vi "Workspace_test.vi"() -> ()   [LabVIEW 2017]
uses:
  NationalInstruments.VeriStand.SystemStorageUI
  NationalInstruments.VeriStand.SystemStorage
  <vilib>/NI Veristand/Execution/Workspace/NI VeriStand - Get Multiple Channel Values.vi
  <vilib>/NI Veristand/Execution/Workspace/NI_VS Workspace ExecutionAPI.lvlib
  <vilib>/NI Veristand/UI Controls/Single Node Browser/NI_VS UI Single Node Browser.lvlib
panel:
  in  "Stop":bool
  in  "NIVS.System Definition Root":refnum<k24>
  in  "Tree Browser":refnum<k24>(container)
  in  "NIVS.Project File Path":path
  in  "Single Node Browser":refnum<k24>(container)
  in  "NIVS.Workspace Event":refnum<event-registration>
  out "System Times":dbl[](array[numeric]) format="%<%H:%M:%S%3u>t"
  out "Targets":string[](array[string])
  in  "NIVS.Gateway IP Address":string
  in  "NIVS.INI File Path":path
  # "Use this example as a template to create custom tools for the NI VeriStand Workspace. This example shows the use of the NI VeriStand API and UI controls to set and get data.\n\nRun this example by adding this VI as a Workspace Tool item. For Help adding Workspace Tool items, please reference the NI VeriStand Help."
  # "With the assistance of the NI VeriStand Execution API, a tool has access to streaming data running on the target."
  # "This is the file path to the VeriStand system definition file. You can read or write to the file using the System Definition API."
  # "This is the root reference to the active System Definition file. You could use this to read the configuration or populate a tree with channels. You are free to close this reference, but it will be closed for you if you don't."
  # "The SystemStorageUI .NET assembly provides controls to display data configured in the System Definition file."
  # "This is the IP Address of the VeriStand Gateway to which the Workspace is connected. Use this to open all the .NET Manager references. Usually the Gateway is running on localhost, but it could be running on a neighbor's machine."
  # "This registered string User Event is used to help instruct your tool to shut down when the Workspace is closing."
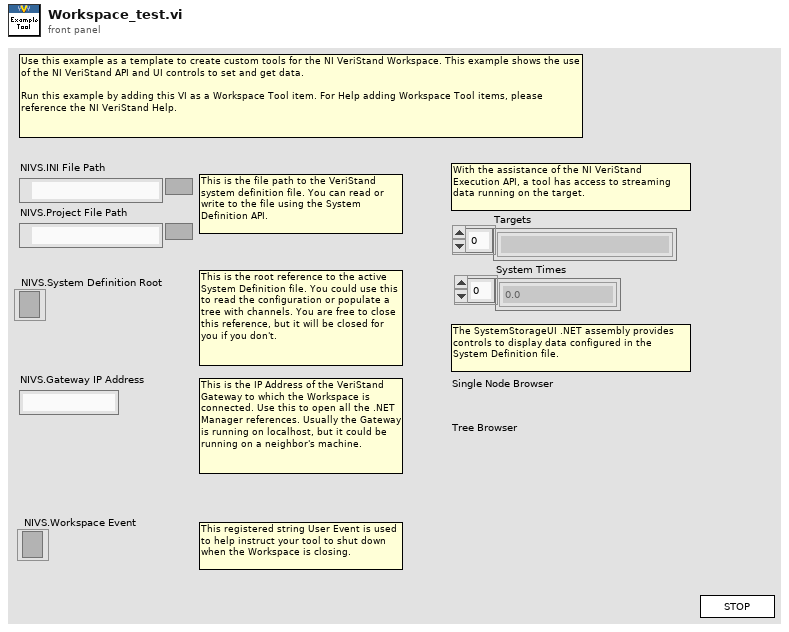
[diagram p1: front panel]
types:
  T1 = typedef "NI_VS UI Single Node Browser.lvlib/Callback Type.ctl" = cluster{"Net Callbacks":refnum<k27>[], "Event":refnum<user-event>}
  T2 = typedef "NI_VS Workspace ExecutionAPI.lvlib/WorkspaceAPI.ctl" = refnum<k24>
  T3 = typedef "NI_VS Workspace ExecutionAPI.lvlib/SystemStateEventRef.ctl" = cluster{"CustDatRef":refnum<user-event>, "EvtRef":refnum<k27>, "Target State User Event":refnum<user-event>}
  T4 = typedef "NI_VS Workspace ExecutionAPI.lvlib/SystemStateRegEventRef.ctl" = refnum<event-registration>
  T5 = cluster{"NIVS.Workspace Event":refnum<event-registration>, "Event Registration Refnum":refnum<event-registration>, "SystemChangeEventRef":T4}
  T6 = typedef "NI_VS UI Single Node Browser.lvlib/Node Ref.ctl" = refnum<k24>
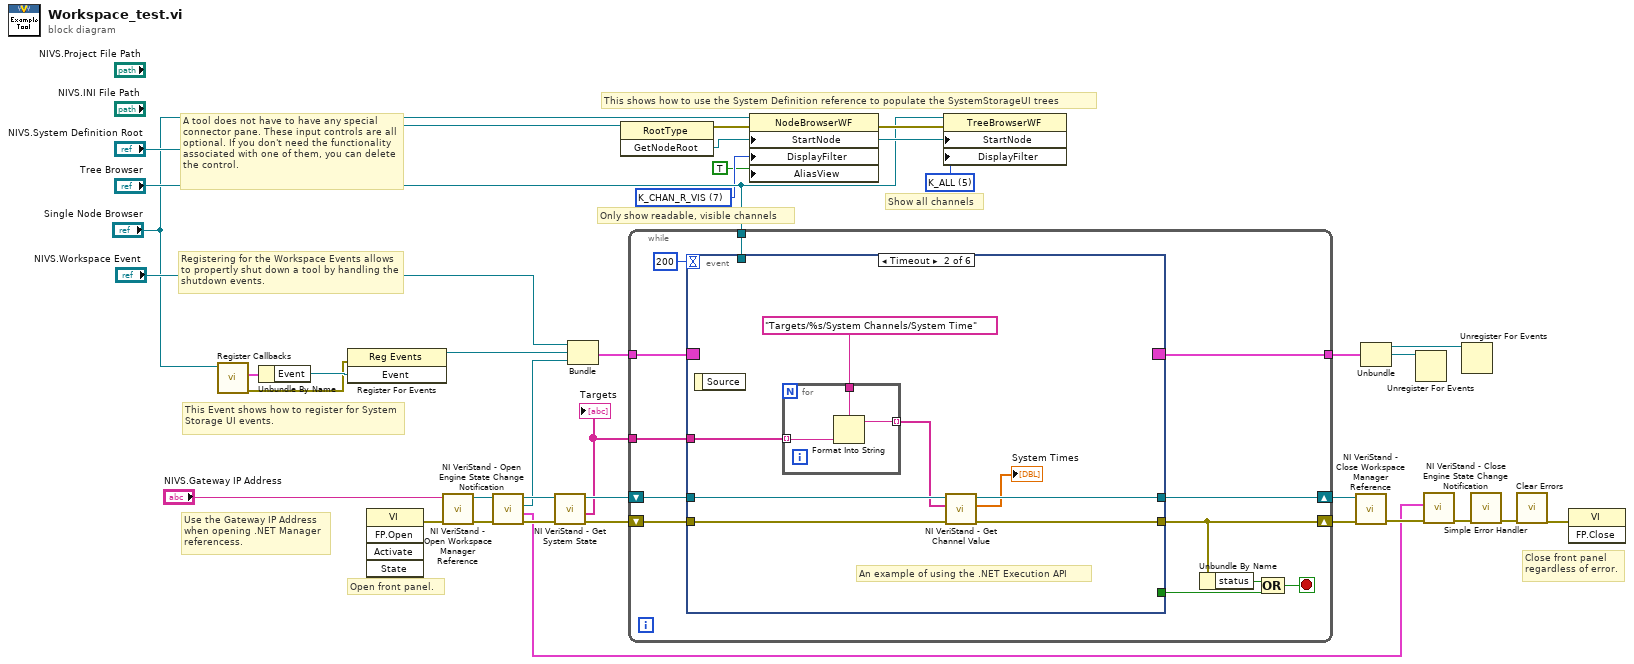
[diagram p0: block diagram]
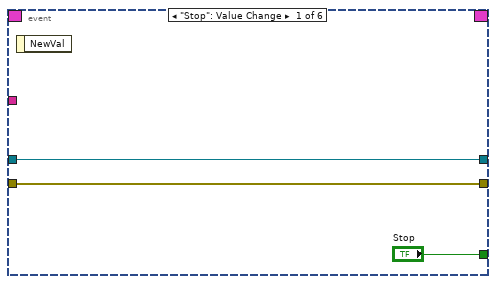
[diagram p2: hidden frame]
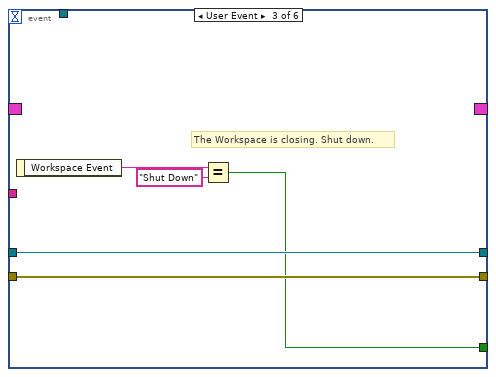
[diagram p3: hidden frame]
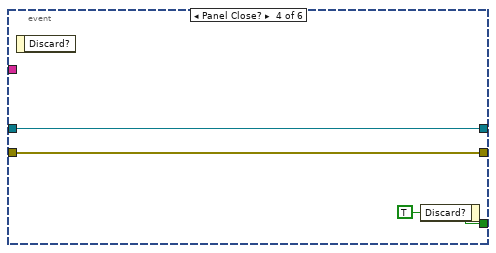
[diagram p4: hidden frame]
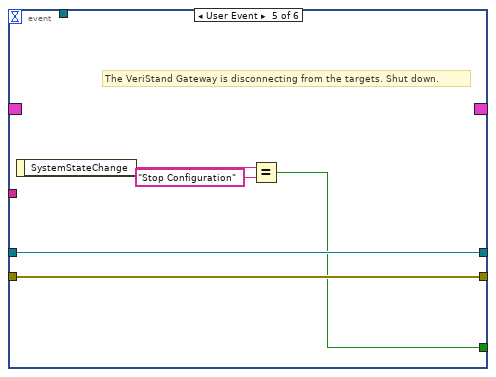
[diagram p5: hidden frame]
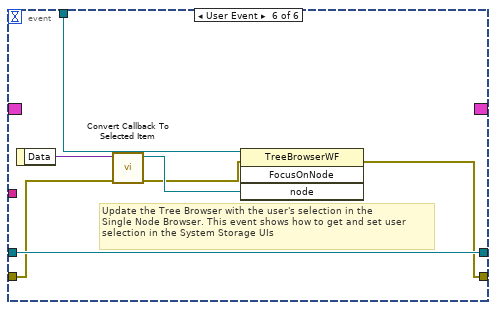
[diagram p6: hidden frame]
diagram:
  w6 = u8 7 items=["K_CHAN_R", "K_CHAN_W", "K_CHAN_RW", "K_CHAN_VOLT", "K_CHAN_FAULT", "K_ALL", "K_CUSTOM", "K_CHAN_R_VIS", "K_CHAN_W_VIS", "K_CHAN_RW_VIS", "K_CHAN_VOLT_VIS", "K_CHAN_FAULT_VIS"] ("DisplayFilter")
  w7 = u8 5 items=["K_CHAN_R", "K_CHAN_W", "K_CHAN_RW", "K_CHAN_VOLT", "K_CHAN_FAULT", "K_ALL", "K_CUSTOM", "K_CHAN_R_VIS", "K_CHAN_W_VIS", "K_CHAN_RW_VIS", "K_CHAN_VOLT_VIS", "K_CHAN_FAULT_VIS"] ("DisplayFilter")
  # "Show all channels"
  # "Only show readable, visible channels"
  # "This Event shows how to register for System Storage UI events."
  # "Use the Gateway IP Address when opening .NET Manager referencess."
  # "A tool does not have to have any special connector pane. These input controls are all optional. If you don't need the functionality associated with one of them, you can delete the control."
  # "This shows how to use the System Definition reference to populate the SystemStorageUI trees"
  # "Registering for the Workspace Events allows to propertly shut down a tool by handling the shutdown events."
  # "Close front panel\nregardless of error."
  # "Open front panel."
  n1 = call <vilib>:"Register Callbacks.vi"("Single Node Browser"="Single Node Browser") -> ("error out"=w1:errorcluster, "Callbacks"=w3:T1)  [unwired: 8 in, 1 out]
  n2 = Unbundle By Name(w3) -> ("Event"=w2:refnum<user-event>)
  n3 = register-events(error in=w1, w2) -> (reference out=w10:refnum<event-registration>)  [unwired: 1 in, 1 out]
  n4 = invoke class="VI" method="FP.Open"() -> (error out=w18:errorcluster)  [unwired: 5 in, 4 out]
  n5 = call <vilib>:"NI VeriStand - Open Workspace Manager Reference.vi"("error in (no error)"=w18, "Gateway IP Address (\"\": localhost)"="NIVS.Gateway IP Address") -> ("error out"=w29:errorcluster, "WorkspaceManager"=w30:T2)  [unwired: 8 in]
  n6 = call <vilib>:"NI VeriStand - Open Engine State Change Notification.vi"("error in (no error)"=w29, "WorkspaceManager in"=w30) -> ("error out"=w34:errorcluster, "SystemStateRefs"=w23:T3, "SystemChangeEventRef"=w9:T4, "WorkspaceManager out"=w35:T2)  [unwired: 6 in]
  n7 = call <vilib>:"NI VeriStand - Get System State.vi"("error in (no error)"=w34, "WorkspaceManager in"=w35) -> ("error out"=w21:errorcluster, "Targets"=w20:string[], "WorkspaceManager  out"=w22:T2)  [unwired: 5 in, 2 out]
  "Targets" <- w20
  n8 = Bundle("NIVS.Workspace Event"="NIVS.Workspace Event", "Event Registration Refnum"=w10, "SystemChangeEventRef"=w9) -> (w28:T5)  [unwired: 1 in]
  n9 = invoke class="RootType" method="GetNodeRoot"(reference="NIVS.System Definition Root") -> (error out=w12:errorcluster, "GetNodeRoot"=w13:refnum<k24>)  [unwired: 2 in, 1 out]
  n10 = while {
    tunnel: w28 -> [w47]
    tunnel: [w46] -> w27
    shift-right: [w39] -> w31
    shift-left: w21 -> [w44]
    shift-right: [w43] -> w32
    shift-left: w22 -> [w45]
    tunnel: w20 -> [w41]
    tunnel: "Tree Browser" -> [w36]
    stop <- w37 stop-if-true
    n11 = event shown="[1] Timeout" {
      selector: w47 -> [_ _ _ _ _ _]
      dyn-events: [_ _ _ _ _ _] -> w46
      timeout: 200 -> [_ _ _ _ _ _]
      tunnel: ["Stop" _ w62 w67 w70 _] -> w38
      tunnel: w45 -> [w49 w58 w65 w68 w73 w81]
      tunnel: w44 -> [w50 w57 w66 w69 w74 w77]
      tunnel: [w50 w52 w66 w69 w74 w75] -> w39
      tunnel: [w49 w53 w65 w68 w73 w81] -> w43
      tunnel: w41 -> [_ w56 _ _ _ _]
      tunnel: w36 -> [_ _ _ _ _ w80]
      event "Stop": Value Change {
        n12 = event-data() -> ()  [unwired: 1 in, 1 out]
      }
      event Timeout {
        # "An example of using the .NET Execution API"
        n13 = event-data() -> ()  [unwired: 1 in, 1 out]
        n14 = for {
          tunnel: w56 -> [w60] mode=indexing
          tunnel: "Targets/%s/System Channels/System Time" ("format string") -> [w61]
          tunnel: [w59] -> w54 mode=indexing
          n15 = Format Into String(format string=w61, w60) -> (resulting string=w59:string)  [unwired: 2 in, 1 out]
        }
        n16 = call-poly <vilib>:"NI VeriStand - Get Channel Value.vi"("error in (no error)"=w57, "Channels"=w54, "WorkspaceManager in"=w58) -> ("error out"=w52:errorcluster, "Values"=→"System Times":dbl[], "WorkspaceManager out"=w53:T2)  [unwired: 6 in]
      }
      event User Event {
        # "The Workspace is closing. Shut down."
        n17 = event-data() -> ("Workspace Event"=w64:string)  [unwired: 1 in]
        n18 = Equal?(x=w64, y="Shut Down") -> (x = y?=w62:bool)
      }
      event Panel Close? {
        w67 = TRUE ("Discard?")
        n19 = event-data() -> ()  [unwired: 1 in, 1 out]
        n20 = event-data("Discard?"=w67) -> ()  [unwired: 1 in, 1 out]
      }
      event User Event {
        # "The VeriStand Gateway is disconnecting from the targets. Shut down."
        n21 = event-data() -> ("SystemStateChange"=w72:string)  [unwired: 1 in]
        n22 = Equal?(x=w72, y="Stop Configuration") -> (x = y?=w70:bool)
      }
      event User Event {
        # "Update the Tree Browser with the user's selection in the\nSingle Node Browser. This event shows how to get and set user\nselection in the System Storage UIs"
        n23 = event-data() -> ("Data"=w79:variant)  [unwired: 1 in]
        n24 = call <vilib>:"Convert Callback To Selected Item.vi"("error in"=w77, "Data"=w79) -> ("error out"=w76:errorcluster, "Selected Item"=w78:T6)  [unwired: 8 in]
        n25 = invoke class="TreeBrowserWF" method="FocusOnNode"(reference=w80, error in=w76, "node"=w78) -> (error out=w75:errorcluster)  [unwired: 1 in, 3 out]
      }
    }
    n26 = Unbundle By Name(w39) -> ("status"=w40:bool)
    n27 = Compound Arithmetic op=OR(w40, w38) -> (w37:bool)
  }
  n28 = property class="NodeBrowserWF"(reference="Single Node Browser", error in=w12, "StartNode"=w13, "DisplayFilter"=w6, "AliasView"=TRUE) -> (error out=w14:errorcluster)  [unwired: 1 out]
  n29 = property class="TreeBrowserWF"(reference="Tree Browser", error in=w14, "StartNode"=w13, "DisplayFilter"=w7) -> ()  [unwired: 2 out]
  n30 = call <vilib>:"NI VeriStand - Close Workspace Manager Reference.vi"("error in (no error)"=w31, "WorkspaceManager"=w32) -> ("error out"=w24:errorcluster)  [unwired: 9 in]
  n31 = Unbundle(w27) -> ("NIVS.Workspace Event"=w25:refnum<event-registration>, "Event Registration Refnum"=w26:refnum<event-registration>)  [unwired: 1 out]
  n32 = Unregister For Events(event registration refnum=w26) -> ()  [unwired: 1 in, 1 out]
  n33 = call <vilib>:"NI VeriStand - Close Engine State Change Notification.vi"("error in (no error)"=w24, "SystemStateRefs"=w23) -> ("error out"=w17:errorcluster)  [unwired: 9 in]
  n34 = Unregister For Events(event registration refnum=w25) -> ()  [unwired: 1 in, 1 out]
  n35 = call <vilib>:"Simple Error Handler.vi"("error in (no error)"=w17) -> ("error out"=w16:errorcluster)  [unwired: 4 in, 4 out]
  n36 = call <vilib>:"Clear Errors.vi"("error in (no error)"=w16) -> ("error out"=w15:errorcluster)  [unwired: 5 in, 1 out]
  n37 = invoke class="VI" method="FP.Close"(error in=w15) -> ()  [unwired: 2 in, 3 out]
